vi "UndoRedo.vi"(7 "Undo (T)":bool=TRUE, 8 "error in (no error)":errorcluster, 9 "editor refs":refnum<vi>[](array[refnum]), 10 "Tree":refnum<vi>, 11 "UndoBuffer":refnum<vi>[](array[refnum])) -> (0 "error out":errorcluster)   [LabVIEW 2020, in "ScriptManager.lvlib"]
uses:
  ScriptManager.lvlib
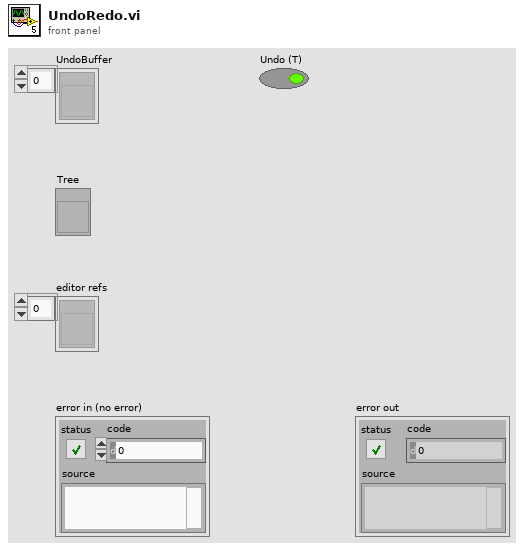
[diagram p1: front panel]
types:
  T1 = cluster{"UndoBuffer[0]":refnum<vi>, "UndoBuffer[1]":refnum<vi>, "UndoBuffer[2]":refnum<vi>}
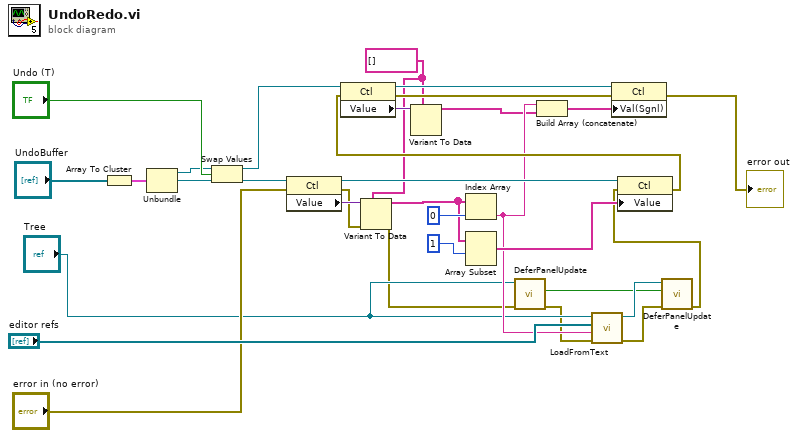
[diagram p0: block diagram]
diagram:
  w9 = string[] []
  n1 = Array To Cluster(array="UndoBuffer") -> (cluster=w29:T1)
  n2 = Unbundle(w29) -> ("UndoBuffer[0]"=w15:refnum<vi>, "UndoBuffer[1]"=w14:refnum<vi>)  [unwired: 1 out]
  n3 = Swap Values(12:w15, 13:"Undo (T)", 14:w14) -> (1:w13:refnum<vi>, 3:w12:refnum<vi>)
  n4 = property class="Ctl"(reference=w12, error in="error in (no error)") -> (reference out=w26:refnum<vi>, error out=w6:errorcluster, "Value"=w28:variant)
  n5 = Variant To Data(error in=w6, type=w9, Variant=w28) -> (data=w11:string[], error out=w5:errorcluster)
  n6 = Index Array(array=w11, index=0) -> (element=w18:string)
  n7 = Array Subset(array=w11, index=1 ("length")) -> (w27:string[])  [unwired: 1 in]
  n8 = call "DeferPanelUpdate.vi"("error in (no error)"=w5, "Control in"="Tree") -> ("error out"=w7:errorcluster, "Defer Panel Updates Old"=w1:bool)  [unwired: 7 in, 1 out]
  n9 = call "LoadFromText.vi"("error in"=w7, "String"=w18, "editor refs"="editor refs", "Tree ref"="Tree") -> ("error out"=w4:errorcluster, "Tree ref out"=w2:refnum<vi>)  [unwired: 6 in]
  n10 = call "DeferPanelUpdate.vi"("error in (no error)"=w4, "Defer Panel Updates (T)"=w1, "Control in"=w2) -> ("error out"=w3:errorcluster)  [unwired: 6 in, 2 out]
  n11 = property class="Ctl"(reference=w26, error in=w3, "Value"=w27) -> (error out=w23:errorcluster)  [unwired: 1 out]
  n12 = property class="Ctl"(reference=w13, error in=w23) -> (reference out=w21:refnum<vi>, error out=w22:errorcluster, "Value"=w20:variant)
  n13 = Variant To Data(type=w9, Variant=w20) -> (data=w10:string[])  [unwired: 1 in, 1 out]
  n14 = Build Array (concatenate)(w18, w10) -> (w19:string[])
  n15 = property class="Ctl"(reference=w21, error in=w22, "Val(Sgnl)"=w19) -> (error out=→"error out":errorcluster)  [unwired: 1 out]
